vi "Day 3 - Mull It Over.vi"() -> ()   [LabVIEW 2020, in "AoC 2024.lvlib"]
uses:
  AoC 2024.lvlib
  <vilib>/regexp/Match Regular Expression.xnode
panel:
  out "Array 2":cluster{i32, i32}[](array[cluster])
  out "Array":cluster{i32, i32}[](array[cluster])
  out "Puzzle Part-2 Answer":string
  out "Puzzle Answer":string
  in  "Puzzle Input":string="xmul(2,4)%&mul[3,7]!@^do_not_mul(5,5)+mul(32,64]then(mul(11,8)mul(8,5))"
  # "Enter the Puzzle Input and run the VI"
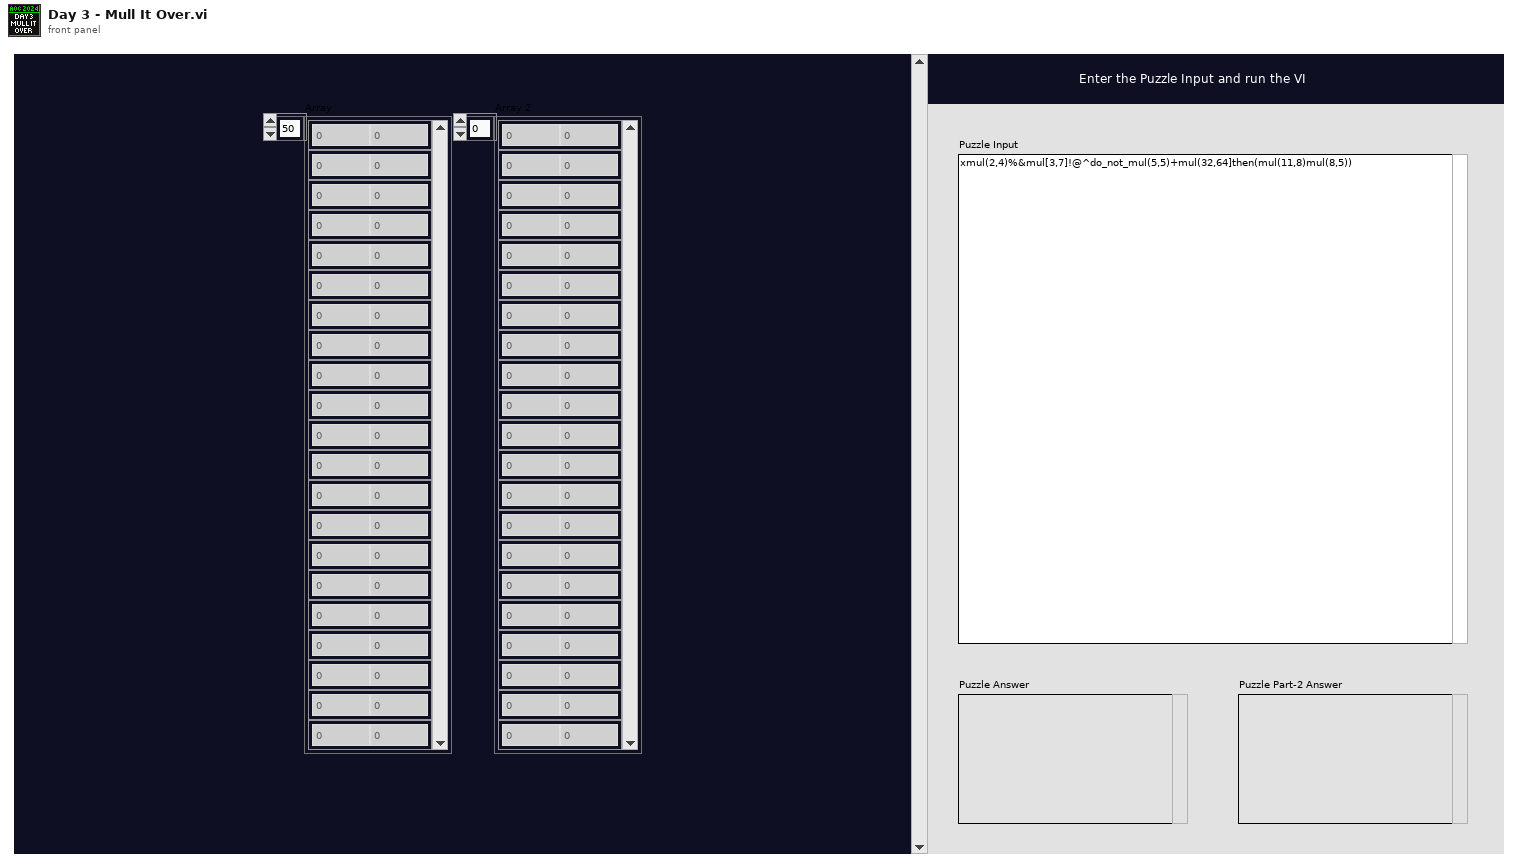
[diagram p1: front panel]
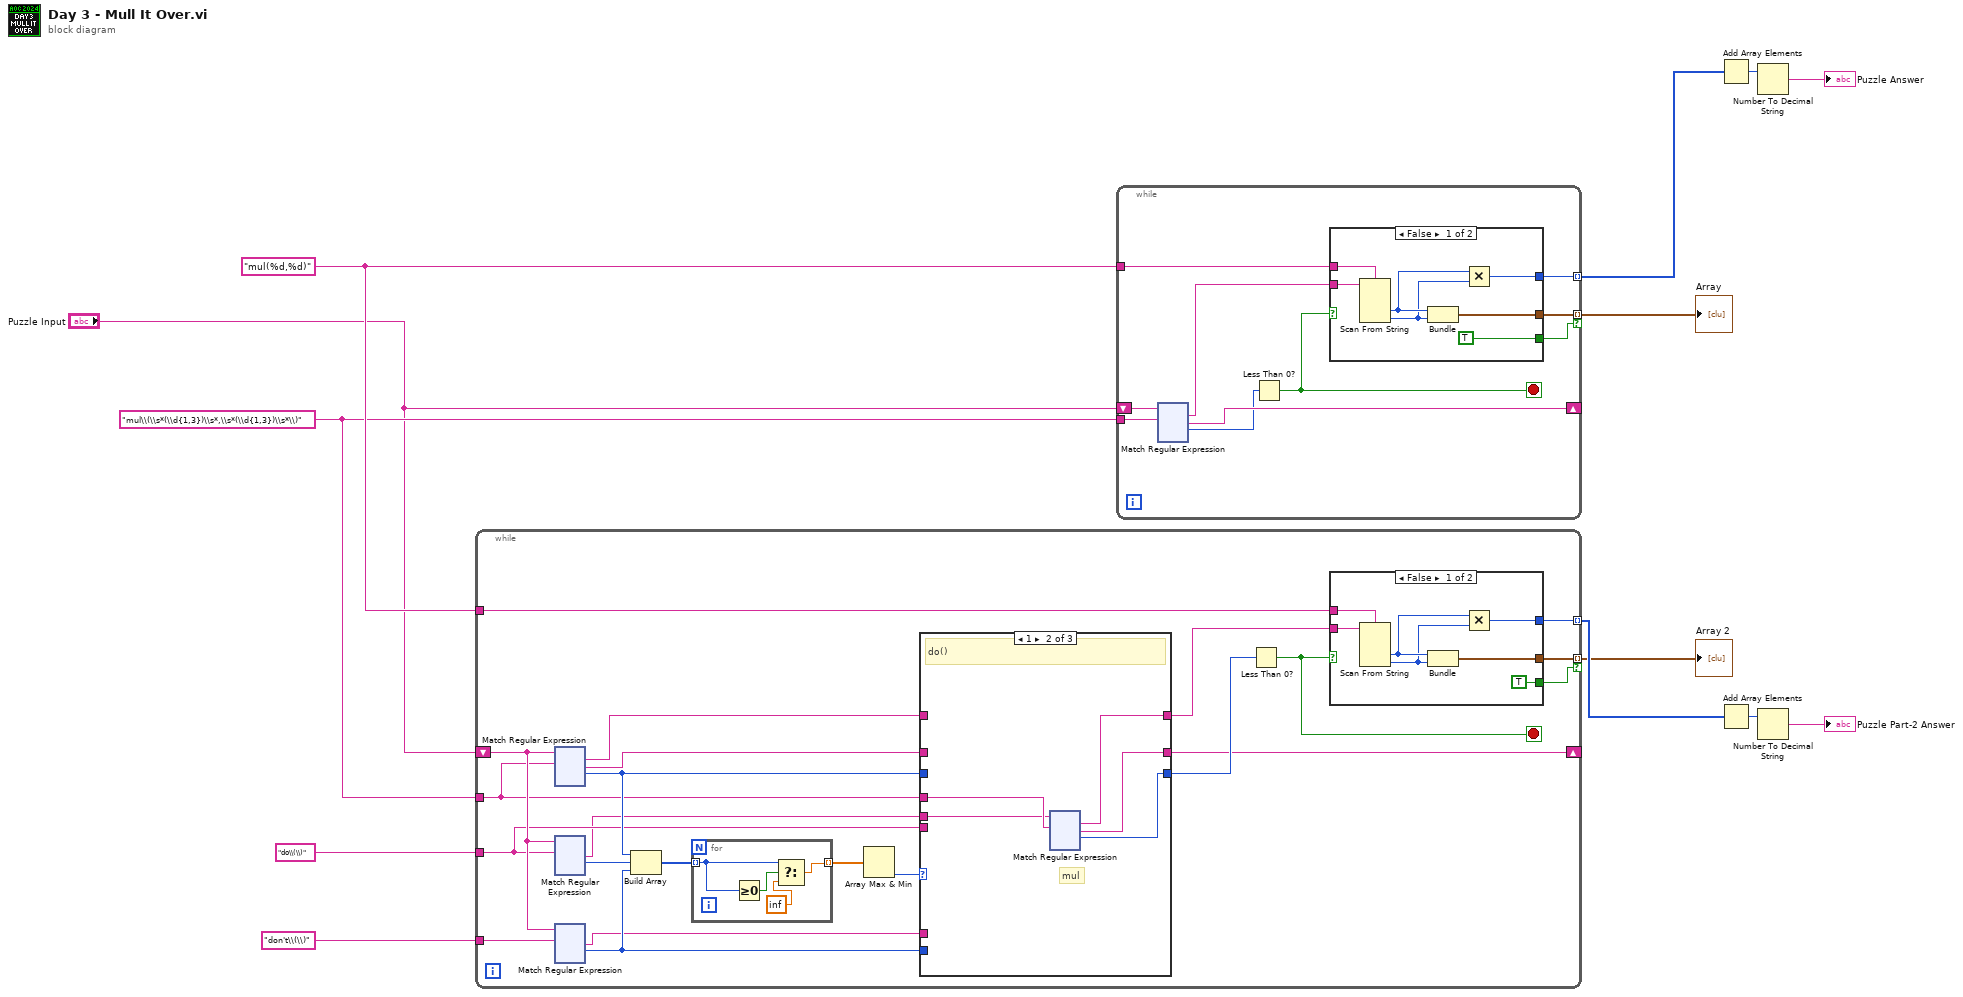
[diagram p0: block diagram]
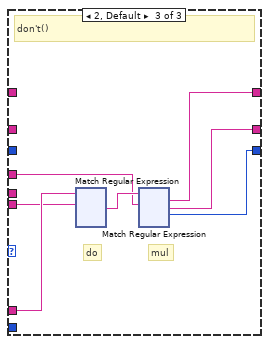
[diagram p3: hidden frame]
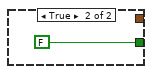
[diagram p4: hidden frame]
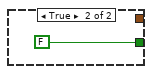
[diagram p5: hidden frame]
diagram:
  w7 = "mul(%d,%d)" ("format string")
  w6 = "mul\\(\\s*(\\d{1,3})\\s*,\\s*(\\d{1,3})\\s*\\)" ("format string")
  n1 = while {
    shift-right: [w26] -> _
    shift-left: "Puzzle Input" -> [w32]
    tunnel: w7 -> [w35]
    tunnel: [w34] -> w2 mode=indexing
    tunnel: w6 -> [w19]
    tunnel: "do\\(\\)" ("format string") -> [w22]
    tunnel: "don't\\(\\)" ("format string") -> [w31]
    tunnel: [w17] -> w1 mode=indexing if=w16
    stop <- w33 stop-if-true
    n2 = xnode "Match Regular Expression"("input string"=w32, "regular expression"=w19) -> ("whole match"=w20:string, "after match"=w25:string, "offset past match"=w28:i32)  [unwired: 4 in, 2 out]
    n3 = xnode "Match Regular Expression"("input string"=w32, "regular expression"=w22) -> ("after match"=w18:string, "offset past match"=w30:i32)  [unwired: 4 in, 3 out]
    n4 = xnode "Match Regular Expression"("input string"=w32, "regular expression"=w31) -> ("after match"=w23:string, "offset past match"=w24:i32)  [unwired: 4 in, 3 out]
    n5 = Build Array(w28, w30, w24) -> (w15:i32[])
    n6 = for {
      tunnel: w15 -> [w38] mode=indexing
      tunnel: [w37] -> w14 mode=indexing
      n7 = Greater Or Equal To 0?(x=w38) -> (x >= 0?=w39:bool)
      n8 = Select(t=w38, s=w39, f=inf) -> (s? t:f=w37:dbl)
    }
    n9 = Array Max & Min(array=w14) -> (min index (indices)=w29:i32)  [unwired: 3 out]
    n10 = case shown="1" w29 {
      tunnel: w28 -> [w40 _ _]
      tunnel: [w40 w45 w163] -> w27
      tunnel: [w41 w46 w164] -> w26
      tunnel: w25 -> [w41 _ _]
      tunnel: w24 -> [_ _ _]
      tunnel: w23 -> [_ _ w168]
      tunnel: w22 -> [_ _ w167]
      tunnel: [w42 w44 w162] -> w21
      tunnel: w20 -> [w42 _ _]
      tunnel: w19 -> [_ w47 w165]
      tunnel: w18 -> [_ w43 _]
      frame 0 {
        # "mul"
      }
      frame 1 {
        # "mul"
        # "do()"
        n11 = xnode "Match Regular Expression"("input string"=w43, "regular expression"=w47) -> ("whole match"=w44:string, "after match"=w46:string, "offset past match"=w45:i32)  [unwired: 4 in, 2 out]
      }
      frame 2, Default {
        # "mul"
        # "do"
        # "don't()"
        n12 = xnode "Match Regular Expression"("input string"=w168, "regular expression"=w167) -> ("after match"=w166:string)  [unwired: 4 in, 4 out]
        n13 = xnode "Match Regular Expression"("input string"=w166, "regular expression"=w165) -> ("whole match"=w162:string, "after match"=w164:string, "offset past match"=w163:i32)  [unwired: 4 in, 2 out]
      }
    }
    n14 = Less Than 0?(x=w27) -> (x < 0?=w33:bool)
    n15 = case shown="False" w33 {
      tunnel: w35 -> [w745 _]
      tunnel: [w744 _] -> w34
      tunnel: w21 -> [w743 _]
      tunnel: [w740 _] -> w17
      tunnel: [TRUE FALSE] -> w16
      frame False {
        n16 = Scan From String(format string=w745, input string=w743) -> (output 1=w742:i32, output 2=w741:i32)  [unwired: 4 in, 3 out]
        n17 = Bundle(w742, w741) -> (w740:cluster{i32, i32})  [unwired: 1 in]
        n18 = Multiply(x=w742, y=w741) -> (x*y=w744:i32)
      }
      frame True {
      }
    }
  }
  "Array 2" <- w1
  n19 = while {
    tunnel: w6 -> [w754]
    tunnel: [w756] -> w9 mode=indexing if=w748
    shift-right: [w753] -> _
    shift-left: "Puzzle Input" -> [w755]
    tunnel: w7 -> [w751]
    tunnel: [w747] -> w8 mode=indexing
    stop <- w749 stop-if-true
    n20 = xnode "Match Regular Expression"("input string"=w755, "regular expression"=w754) -> ("whole match"=w752:string, "after match"=w753:string, "offset past match"=w750:i32)  [unwired: 4 in, 2 out]
    n21 = Less Than 0?(x=w750) -> (x < 0?=w749:bool)
    n22 = case shown="False" w749 {
      tunnel: [w763 _] -> w756
      tunnel: w752 -> [w762 _]
      tunnel: w751 -> [w761 _]
      tunnel: [TRUE FALSE] -> w748
      tunnel: [w757 _] -> w747
      frame False {
        n23 = Scan From String(format string=w761, input string=w762) -> (output 1=w759:i32, output 2=w758:i32)  [unwired: 4 in, 3 out]
        n24 = Bundle(w759, w758) -> (w763:cluster{i32, i32})  [unwired: 1 in]
        n25 = Multiply(x=w759, y=w758) -> (x*y=w757:i32)
      }
      frame True {
      }
    }
  }
  "Array" <- w9
  n26 = Add Array Elements(numeric array=w8) -> (sum=w11:i32)
  n27 = Add Array Elements(numeric array=w2) -> (sum=w10:i32)
  n28 = Number To Decimal String(number=w11) -> (decimal integer string=→"Puzzle Answer":string)  [unwired: 1 in]
  n29 = Number To Decimal String(number=w10) -> (decimal integer string=→"Puzzle Part-2 Answer":string)  [unwired: 1 in]
